vi "Ramp_Lauda_v3.vi"(0 "manual":i32, 1 "Tr_Tj":i32=1, 2 "shutdown":i32, 3 "S1_S2":i32, 5 "Tr":dbl[](array[numeric]), 6 "T_fail":dbl, 8 "enable":i32, 9 "time_set":dbl[](array[numeric]), 16 "reset":i32, 17 "time_wait":dbl[](array[numeric]), 19 "T_S2":dbl, 20 "port":i32=1, 21 "T_sp":dbl[](array[numeric])) -> (4 "elapsed":dbl, 10 "LED_1":bool, 11 "LED_manual":bool, 12 "LED_2":bool, 13 "T0_":dbl, 14 "step":dbl, 15 "LED_stop":bool, 18 "LED_3":bool, 22 "LED 4":bool, 23 "LED 5":bool, 24 "setpoint":dbl, 25 "Tr_out":dbl, 27 "T int":dbl)   [LabVIEW 2016]
uses:
  BERTTA/x64/Debug/BERTTA.dll
panel:
  out "Count":dbl
  out "Tpause":dbl
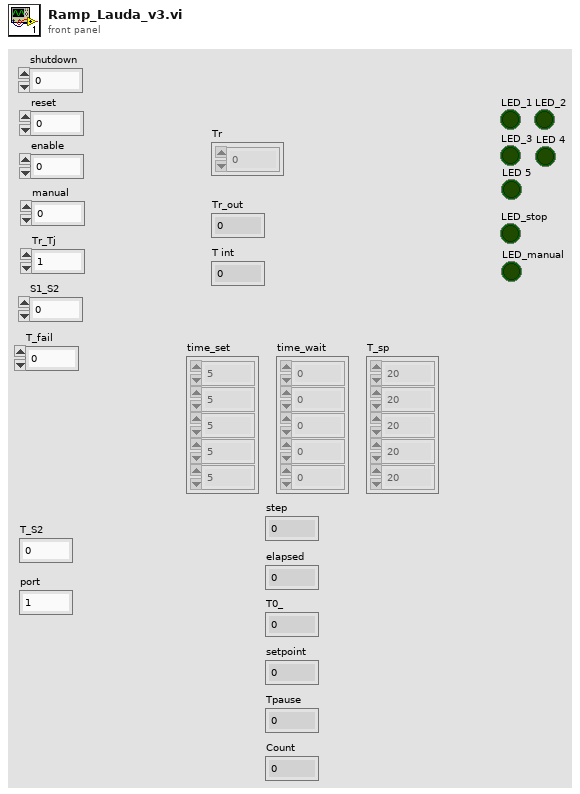
[diagram p1: front panel]
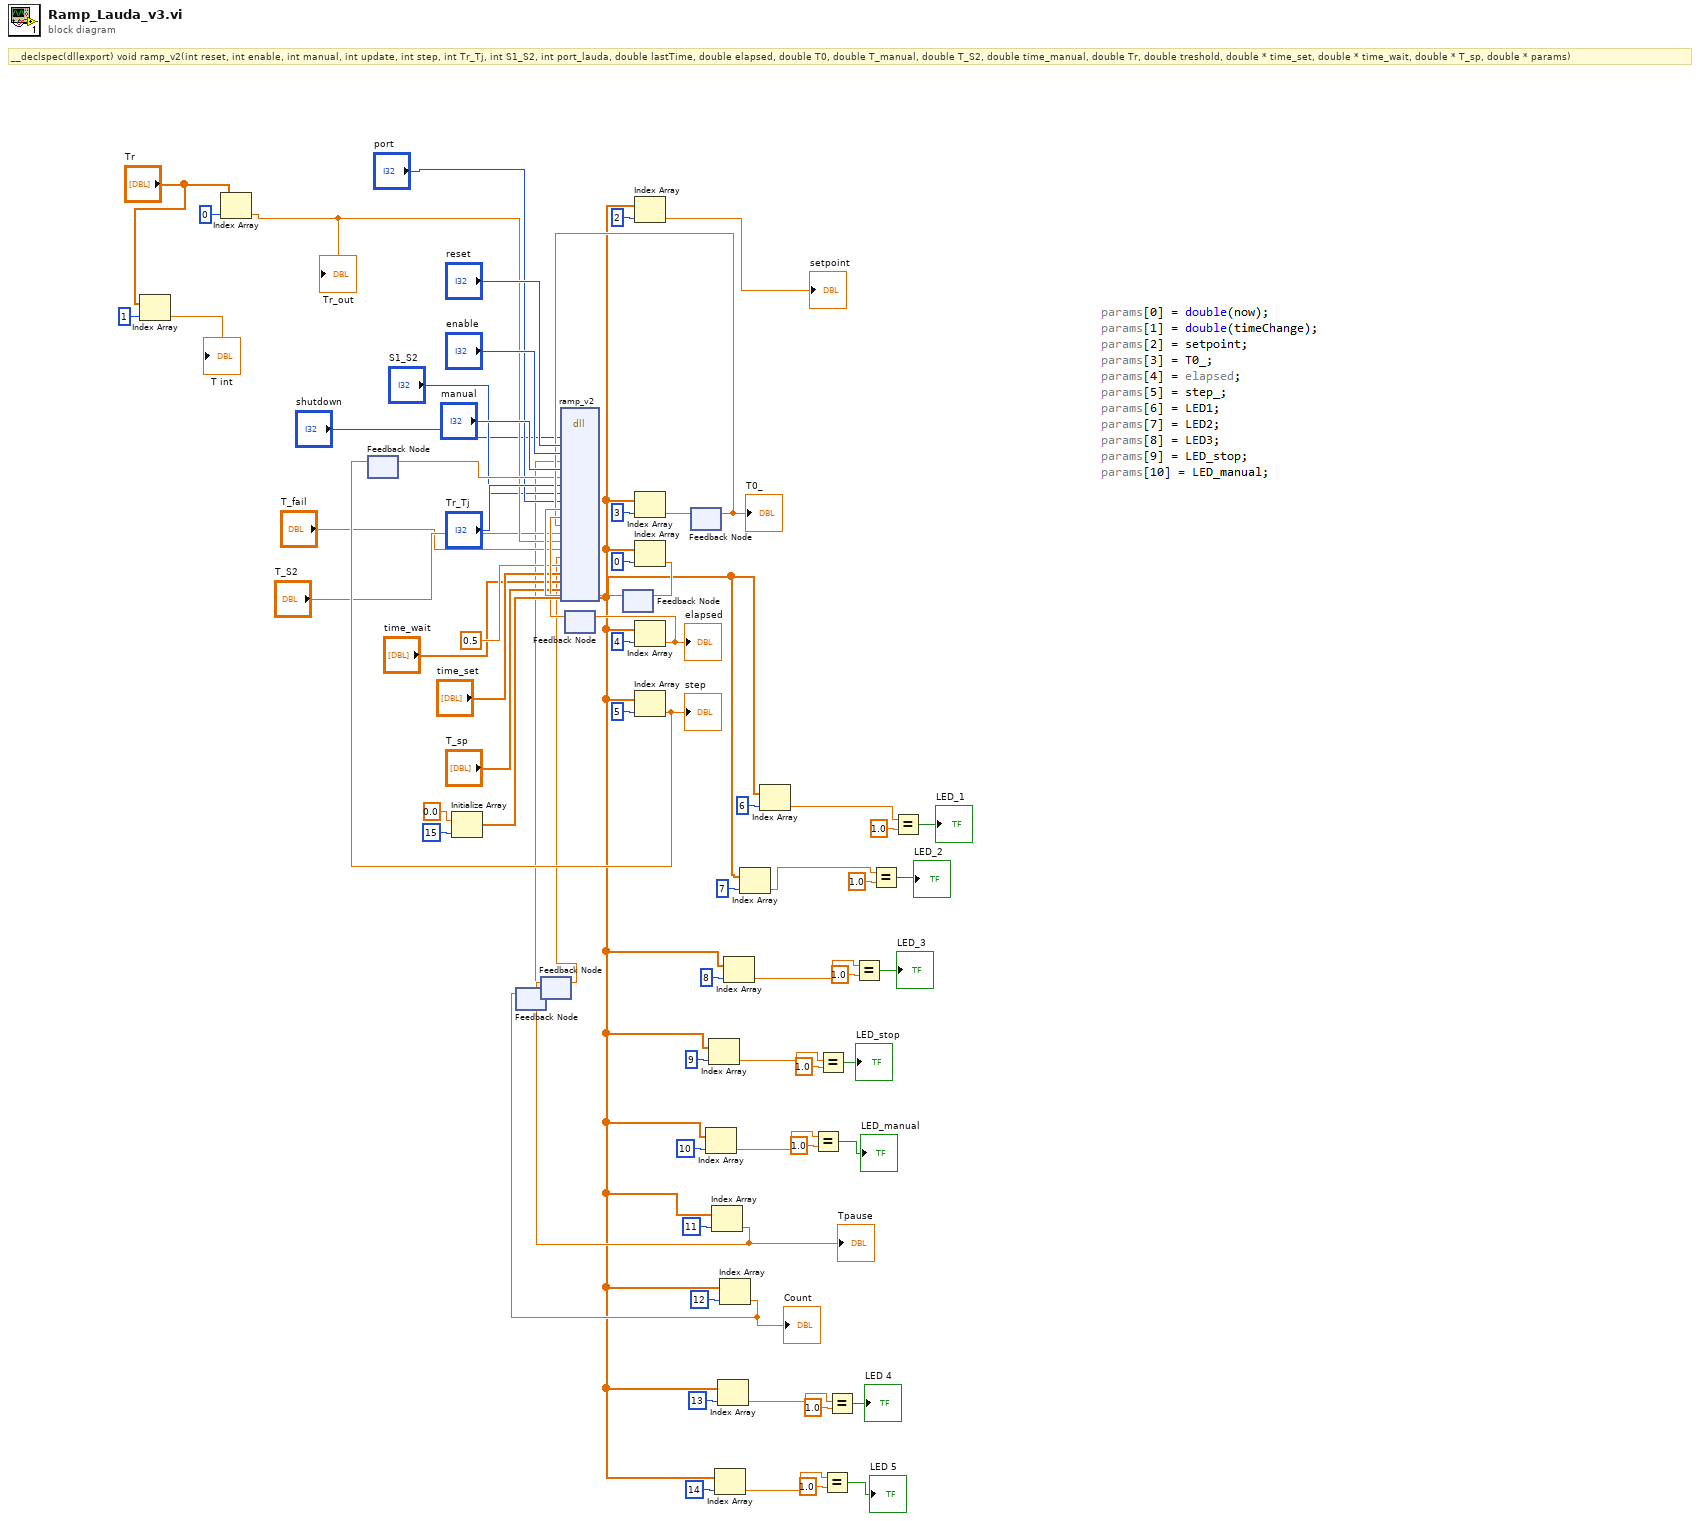
[diagram p0: block diagram]
diagram:
  # "__declspec(dllexport) void ramp_v2(int reset, int enable, int manual, int update, int step, int Tr_Tj, int S1_S2, int port_lauda, double lastTime, double elapsed, double T0, double T_manual, double T_S2, double time_manual, double Tr, double treshold, double * time_set, double * time_wait, double * T_sp, double * params)"
  n1 = Index Array(array="Tr", index=1) -> (element=→"T int":dbl)
  n2 = Index Array(array="Tr", index=0) -> (element=w43:dbl)
  "Tr_out" <- w43
  n3 = feedback #1() -> (w50:dbl)  [unwired: 1 in]
  n4 = Initialize Array(0.0 ("element"), 15 ("dimension size")) -> (w65:dbl[])
  n5 = feedback #2() -> (w11:dbl)  [unwired: 1 in]
  n6 = feedback #3() -> (w14:dbl)  [unwired: 1 in]
  n7 = feedback #4() -> (w59:dbl)  [unwired: 1 in]
  n8 = feedback #5() -> (w62:dbl)  [unwired: 1 in]
  n9 = feedback #6() -> (w56:dbl)  [unwired: 1 in]
  "T0_" <- w56
  n10 = dll-call lib="C:/Users/shresplab/OneDrive - Kemira Oyj/Documents/GitHub/Bertta/BERTTA/x64/Debug/BERTTA.dll" fn="ramp_v2"("shutdown"="shutdown", "reset"="reset", "enable"="enable", "count"=w11, "manual"="manual", "step"=w50, "Tr_Tj"="Tr_Tj", "S1_S2"="S1_S2", "port_lauda"="port", "lastTime"=w62, "elapsed"=w59, "T0"=w56, "T_S2"="T_S2", "Tr"=w43, "T_fail"="T_fail", "Tpause"=w14, "treshold"=0.5, "time_set"="time_set", "time_wait"="time_wait", "T_sp"="T_sp", "params"=w65) -> ("params"=w2:dbl[])  [unwired: 24 in, 2 out]
  n11 = Index Array(array=w2, index=2) -> (element=→"setpoint":dbl)
  n12 = Index Array(array=w2, index=3) -> (element=w57:dbl)
  n13 = Index Array(array=w2, index=0) -> (element=w63:dbl)
  n14 = feedback-in #5(w63) -> ()
  n15 = Index Array(array=w2, index=4) -> (element=w60:dbl)
  "elapsed" <- w60
  n16 = feedback-in #4(w60) -> ()
  n17 = Index Array(array=w2, index=5) -> (element=w51:dbl)
  "step" <- w51
  n18 = feedback-in #1(w51) -> ()
  n19 = feedback-in #6(w57) -> ()
  n20 = Index Array(array=w2, index=10) -> (element=w25:dbl)
  n21 = Index Array(array=w2, index=9) -> (element=w26:dbl)
  n22 = Index Array(array=w2, index=11) -> (element=w15:dbl)
  "Tpause" <- w15
  n23 = feedback-in #3(w15) -> ()
  n24 = Index Array(array=w2, index=14) -> (element=w5:dbl)
  n25 = Index Array(array=w2, index=13) -> (element=w6:dbl)
  n26 = Index Array(array=w2, index=12) -> (element=w12:dbl)
  "Count" <- w12
  n27 = feedback-in #2(w12) -> ()
  n28 = Index Array(array=w2, index=8) -> (element=w27:dbl)
  n29 = Index Array(array=w2, index=7) -> (element=w28:dbl)
  n30 = Index Array(array=w2, index=6) -> (element=w33:dbl)
  n31 = Equal?(x=w25, y=1.0) -> (x = y?=→"LED_manual":bool)
  n32 = Equal?(x=w26, y=1.0) -> (x = y?=→"LED_stop":bool)
  n33 = Equal?(x=w5, y=1.0) -> (x = y?=→"LED 5":bool)
  n34 = Equal?(x=w6, y=1.0) -> (x = y?=→"LED 4":bool)
  n35 = Equal?(x=w27, y=1.0) -> (x = y?=→"LED_3":bool)
  n36 = Equal?(x=w28, y=1.0) -> (x = y?=→"LED_2":bool)
  n37 = Equal?(x=w33, y=1.0) -> (x = y?=→"LED_1":bool)
